vi "Write Complex Data (Format Into String) to File.vi"() -> ()   [LabVIEW 2016]
panel:
  in  "Boolean":bool
  in  "Final String":string
  in  "Voltage":dbl
  in  "Initial String":string
  in  "Format String":string
  in  "Operation on File":T1(ring)
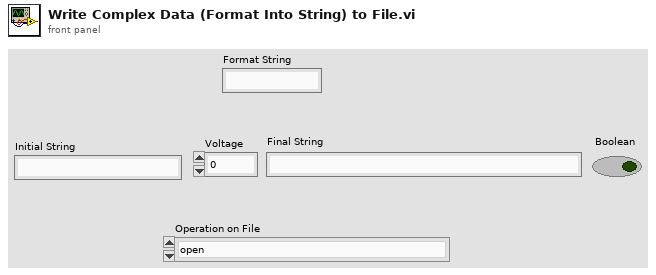
[diagram p1: front panel]
types:
  T1 = enum16{"open", "replace", "create", "open or create", "replace or create", "replace or create with confirmation"}
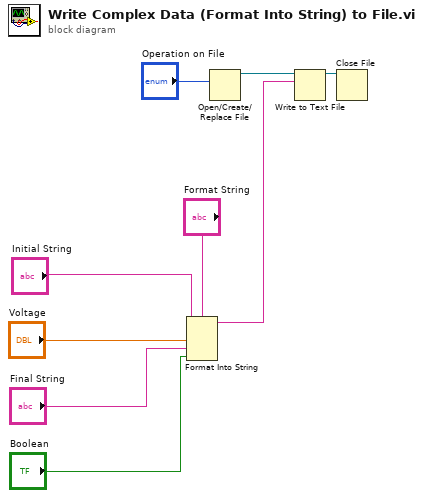
[diagram p0: block diagram]
diagram:
  n1 = Format Into String(format string="Format String", initial string="Initial String", "Voltage", "Final String", "Boolean") -> (resulting string=w1:string)  [unwired: 1 in, 1 out]
  n2 = Open/Create/Replace File(operation (0:open)="Operation on File") -> (refnum out=w9:refnum<file>)  [unwired: 5 in, 2 out]
  n3 = Write to Text File(file (use dialog)=w9, text=w1) -> (refnum out=w8:refnum<file>)  [unwired: 2 in, 2 out]
  n4 = Close File(refnum=w8) -> ()  [unwired: 1 in, 2 out]
